vi "NameMap-Check.vi"(8 "error in (no error)":errorcluster, 10 "Name":string, 11 "NameMap in":T1) -> (0 "error out":errorcluster, 2 "OriginName":string, 3 "NameMap out":T1)   [LabVIEW 2019]
uses:
  Typedef/Def-NameMap.ctl
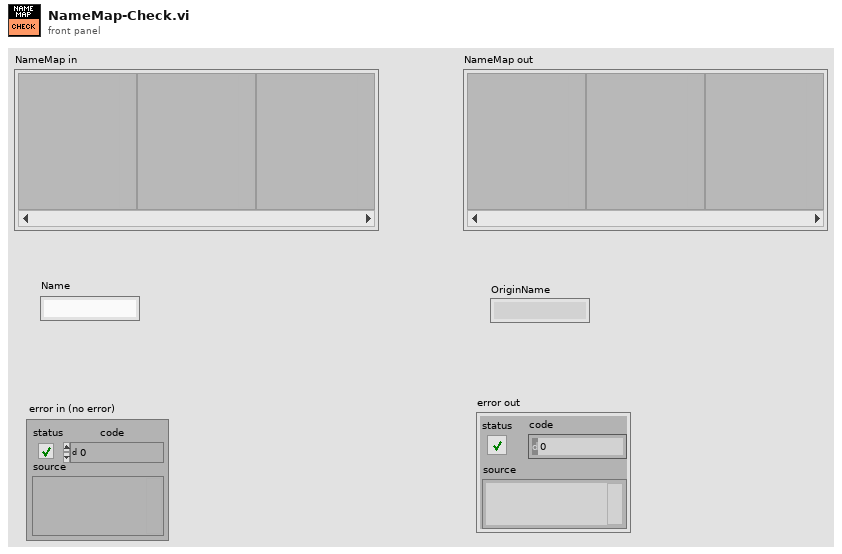
[diagram p1: front panel]
types:
  T1 = typedef "Def-NameMap.ctl" = variant[]
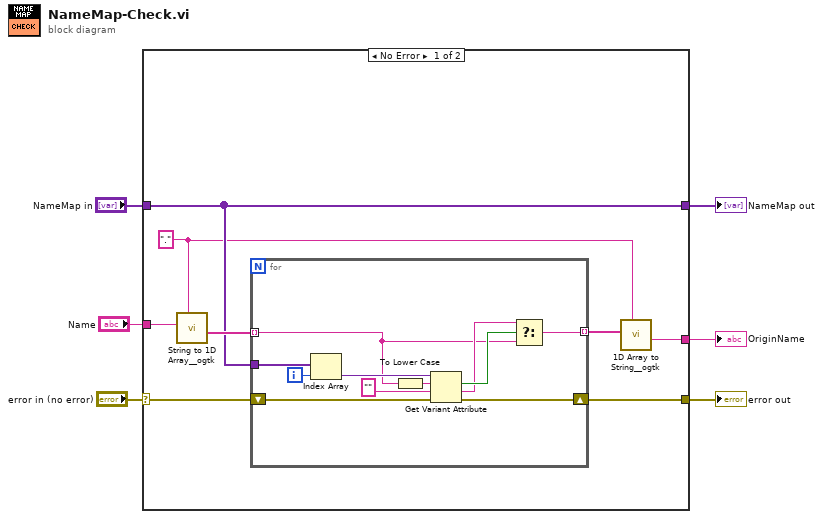
[diagram p0: block diagram]
diagram:
  n1 = case shown="No Error" "error in (no error)" {
    selector: "error in (no error)" -> [w13 w28]
    tunnel: "Name" -> [w14 w26]
    tunnel: [w10 w27] -> w5
    tunnel: [w12 w28] -> w3
    tunnel: "NameMap in" -> [w10 w27]
    tunnel: [w7 w26] -> w1
    frame No Error {
      w8 = "." ("delimiter (Tab)")
      n2 = call <userlib>:"String to 1D Array__ogtk.vi"("delimiter (Tab)"=w8, "string"=w14) -> ("Array of Strings"=w11:string[])  [unwired: 9 in]
      n3 = for {
        tunnel: w11 -> [w16] mode=indexing
        shift-right: [w22] -> w12
        shift-left: w13 -> [w21]
        tunnel: w10 -> [w19]
        tunnel: [w15] -> w9 mode=indexing
        i -> [w25]
        n4 = Index Array(array=w19, index=w25) -> (element=w24:variant)
        n5 = To Lower Case(string=w16) -> (all lower case string=w20:string)
        n6 = Get Variant Attribute(Variant=w24, name=w20, default value (empty Variant)="" ("delimiter (Tab)"), error in=w21) -> (found=w18:bool, value=w17:string, error out=w22:errorcluster)  [unwired: 1 out]
        n7 = Select(t=w17, s=w18, f=w16) -> (s? t:f=w15:string)
      }
      n8 = call <userlib>:"1D Array to String__ogtk.vi"("delimiter (Tab)"=w8, "Array of Strings"=w9) -> ("delimited string"=w7:string)  [unwired: 9 in]
    }
    frame Error {
    }
  }
  "NameMap out" <- w5
  "error out" <- w3
  "OriginName" <- w1
